vi "Periodic Tasks.vi"(8 "error in":errorcluster) -> ()   [LabVIEW 2016]
doc: "This VI runs in parallel to other tasks. It can contain as many user-defined periodic loops as you need. These can carry out PID or other sorts of timed response."
uses:
  Refname/Motors.ctl
  Refname/Sensors.ctl
  Refname/Queues.ctl
  <vilib>/Rock Robotics/WPI/DriverStation/WPI_DriverStationRobotMode2.ctl
  Refname/Refname to String (Motors).vi
  Robot Global Data.vi
  Refname/Refname to String (Sensors).vi
panel:
  in  "Low Sensitivity z":dbl=1.9 format="%#_13g"
  in  "Default Sensitivity z":dbl=1.6 format="%#_13g"
  in  "Low Sensitivity x & y":dbl=1.7 format="%#_13g"
  in  "Default Sensitivity x & y":dbl=1.4 format="%#_13g"
  out "error out":errorcluster
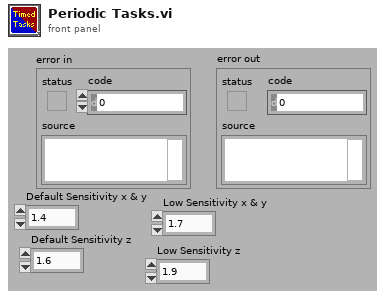
[diagram p1: front panel]
types:
  T1 = typedef "Queues.ctl" = enum16{"Log Queue"}
  T2 = typedef "Sensors.ctl" = enum16{"DIP 1", "DIP 2", "DIP 3", "DIP 4", "IMU", "HuskieBoard"}
  T3 = typedef "Motors.ctl" = enum16{"Wheel 1", "Swerve 1", "Wheel 2", "Swerve 2", "Wheel 3", "Swerve 3", "Wheel 4", "Swerve 4", "Climber"}
  T4 = typedef "WPI_MotorControlDeviceRef.ctl" = cluster{"DeviceStatus":errorcluster, "Type":T5, "PWM":cluster{"PWM Channel":T6, "DeadBand":T7}, "CAN":cluster{"Device Number":u8, "SetOutput VI Ref":variant, "GetOutput VI Ref":variant, "Enable VI Ref":variant, "Disable VI Ref":variant, "Data":variant}, "Invert":bool}
  T5 = typedef "WPI_MotorControlType.ctl" = enum16{"PWM", "CAN"}
  T6 = typedef "FPGA_DIOPWMChannel.ctl" = enum8{"PWM 0", "PWM 1", "PWM 2", "PWM 3", "PWM 4", "PWM 5", "PWM 6", "PWM 7", "PWM 8", "PWM 9", "PWM MXP 0", "PWM MXP 1", "PWM MXP 2", "PWM MXP 3", "PWM MXP 4", "PWM MXP 5", "PWM MXP 6", "PWM MXP 7", "PWM MXP 8", "PWM MXP 9", "Invalid"}
  T7 = typedef "WPI_PWMDeadband.ctl" = cluster{"Name":string, "maxPositivePwm":i32, "minPositivePwm":i32, "centerPwm":i32, "maxNegativePwm":i32, "minNegativePwm":i32, "angularRange":u16}
  T8 = typedef "WPI_SerialPortRef.ctl" = cluster{"DevStatus":errorcluster, "Serial Port Name":refnum<visa-resource-name>}
  T9 = typedef "WPI_DriverStationRobotMode2.ctl" = enum16{"Autonomous Disabled", "Autonomous Enabled", "Teleop Disabled", "Teleop Enabled", "Disconnected", "Finish", "Test Disabled", "Test Enabled", "Emergency Stopped"}
  T10 = cluster{"X":dbl, "Y":dbl, "Z":dbl, "B (Straight Drive)":bool, "T1 (Climber Up)":bool, "T2 (Climber Down)":bool, "Pinky Trigger (Low Sensitivity Drive)":bool, "Trigger Full Press (Reverse Drive)":bool}
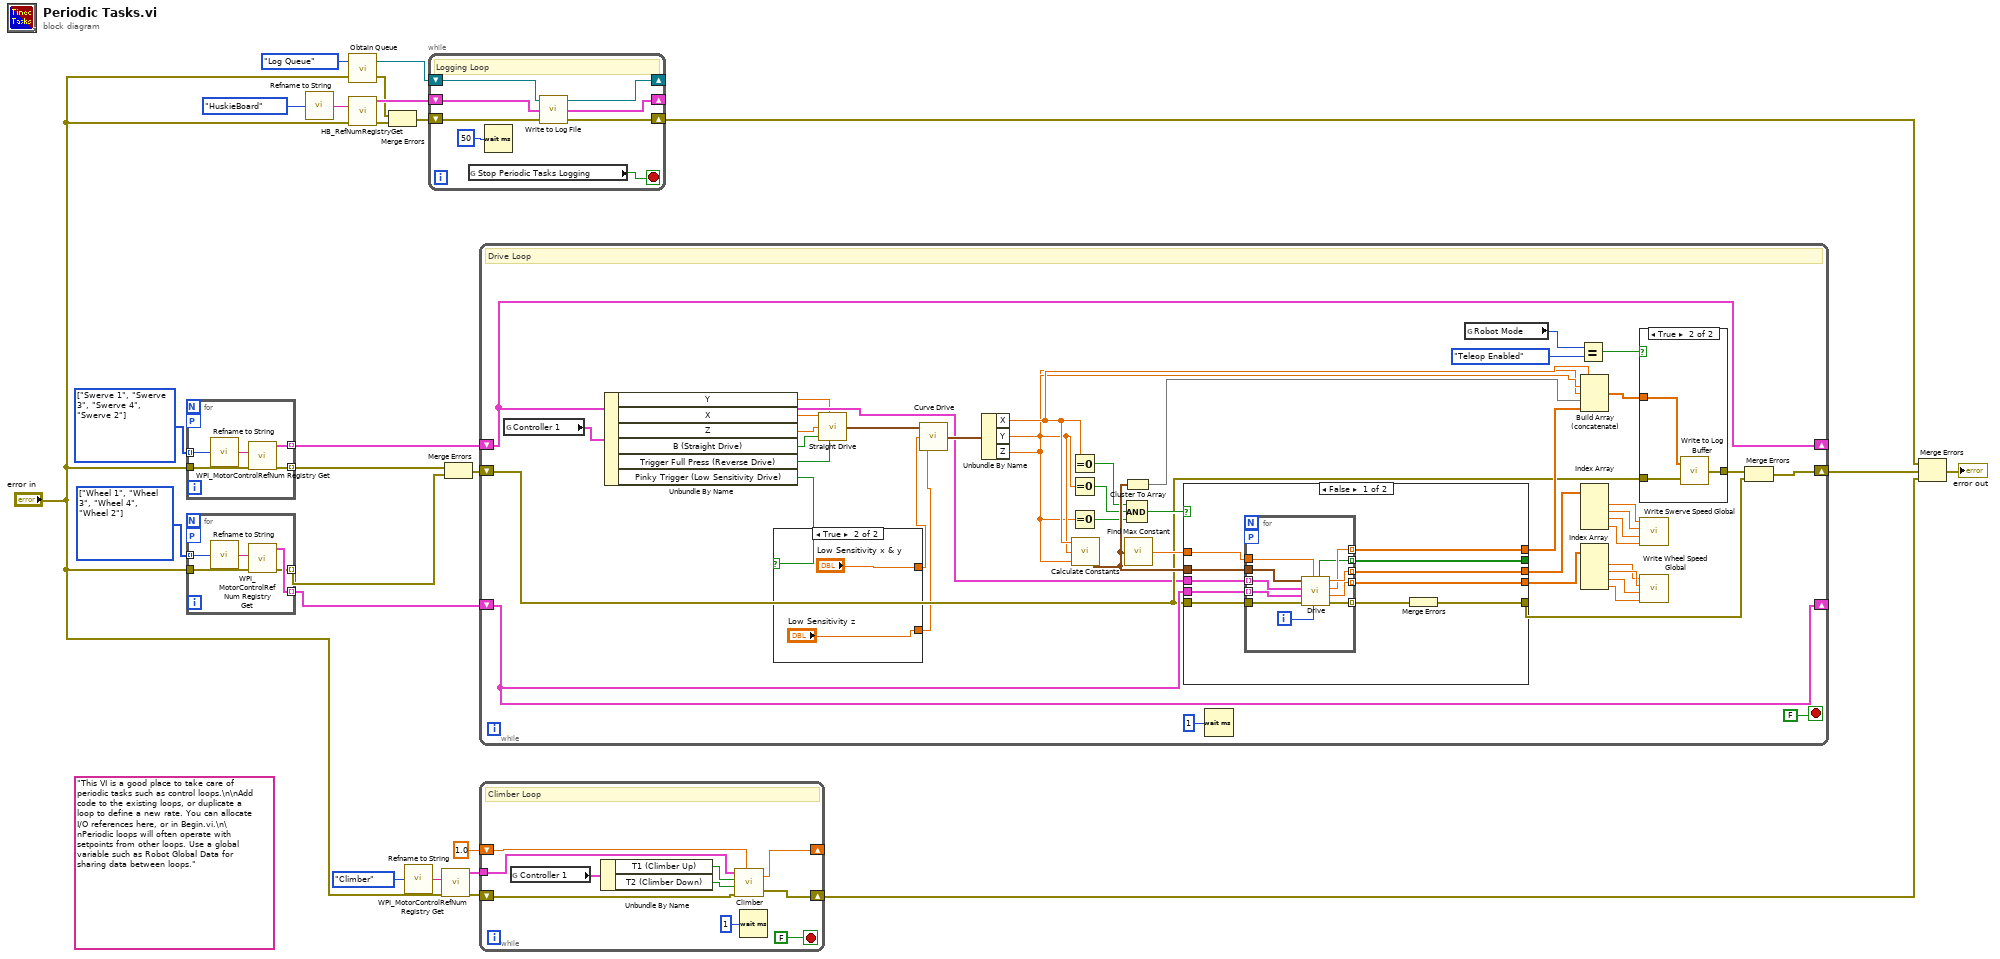
[diagram p0: block diagram]
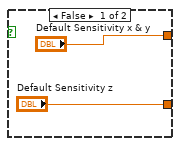
[diagram p2: hidden frame]
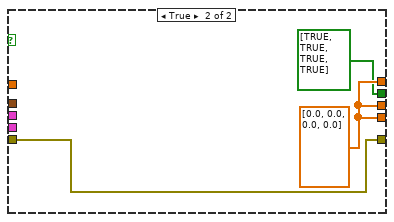
[diagram p3: hidden frame]
diagram:
  w22 = T3[] [enum."Wheel 1", enum."Wheel 3", enum."Wheel 4", enum."Wheel 2"] items=["Wheel 1", "Swerve 1", "Wheel 2", "Swerve 2", "Wheel 3", "Swerve 3", "Wheel 4", "Swerve 4", "Climber"]
  w23 = T3[] [enum."Swerve 1", enum."Swerve 3", enum."Swerve 4", enum."Swerve 2"] items=["Wheel 1", "Swerve 1", "Wheel 2", "Swerve 2", "Wheel 3", "Swerve 3", "Wheel 4", "Swerve 4", "Climber"]
  (unwired) "This VI is a good place to take care of periodic tasks such as control loops.\n\nAdd code to the existing loops, or duplicate a loop to define a new rate. You can allocate I/O references here, or in Begin.vi.\n\nPeriodic loops will often operate with setpoints from other loops. Use a global variable such as Robot Global Data for sharing data between loops."
  n1 = for {
    tunnel: [w30] -> w25 mode=indexing
    tunnel: w23 -> [w28] mode=indexing
    workers-P: _ -> [_]
    tunnel: "error in" -> [w27]
    tunnel: [w26] -> w20 mode=indexing
    n2 = call-poly "Refname to String.vi"("Enum"=w28) -> ("String"=w29:string)
    n3 = call <vilib>:"WPI_MotorControlRefNum Registry Get.vi"("error in (no error)"=w27, "refnum name"=w29) -> ("error out"=w26:errorcluster, "MotorControlDevRef"=w30:T4)  [unwired: 8 in]
  }
  n4 = for {
    tunnel: [w35] -> w24 mode=indexing
    tunnel: w22 -> [w33] mode=indexing
    workers-P: _ -> [_]
    tunnel: "error in" -> [w32]
    tunnel: [w31] -> w19 mode=indexing
    n5 = call-poly "Refname to String.vi"("Enum"=w33) -> ("String"=w34:string)
    n6 = call <vilib>:"WPI_MotorControlRefNum Registry Get.vi"("error in (no error)"=w32, "refnum name"=w34) -> ("error out"=w31:errorcluster, "MotorControlDevRef"=w35:T4)  [unwired: 8 in]
  }
  n7 = call-poly "Refname to String.vi"("Enum"=Sensors."HuskieBoard") -> ("String"=w11:string)
  n8 = call "Obtain Queue.vi"("error in"="error in", "Queue"=Queues."Log Queue") -> ("error out"=w5:errorcluster, "Queue Ref"=w8:refnum<queue>)
  n9 = call <vilib>:"HB_RefNumRegistryGet.vi"("refnum name"=w11, "error in (no error)"="error in") -> ("HBDevRef"=w7:T8, "error out"=w4:errorcluster)  [unwired: 12 in]
  n10 = Merge Errors(w5, w4) -> (w6:errorcluster)
  n11 = call-poly "Refname to String.vi"("Enum"=Motors."Climber") -> ("String"=w18:string)
  n12 = while {
    shift-right: [w41] -> _
    shift-left: w8 -> [w42]
    shift-right: [w39] -> _
    shift-left: w7 -> [w40]
    shift-right: [w37] -> w3
    shift-left: w6 -> [w38]
    stop <- w43 stop-if-true
    # "Logging Loop"
    n13 = global read "Robot Global Data.vi" "Stop Periodic Tasks Logging"() -> (w43:bool)
    n14 = Wait (ms)(milliseconds to wait=u32 50) -> ()  [unwired: 1 out]
    n15 = call "Write to Log File.vi"("error in"=w38, "HBDevRef"=w40, "Log Queue"=w42) -> ("error out"=w37:errorcluster, "HBDevRef"=w39:T8, "Log Queue"=w41:refnum<queue>)
  }
  n16 = call <vilib>:"WPI_MotorControlRefNum Registry Get.vi"("error in (no error)"="error in", "refnum name"=w18) -> ("error out"=w15:errorcluster, "MotorControlDevRef"=w16:T4)  [unwired: 8 in]
  n17 = Merge Errors(w20, w19) -> (w13:errorcluster)
  n18 = while {
    shift-right: [w53] -> _
    shift-left: w25 -> [w53]
    shift-right: [w85] -> _
    shift-left: w24 -> [w85]
    shift-right: [w68] -> w2
    shift-left: w13 -> [w54]
    stop <- FALSE stop-if-true
    # "Drive Loop"
    n19 = global read "Robot Global Data.vi" "Controller 1"() -> (w49:T10)
    n20 = Unbundle By Name(w49) -> ("Y"=w45:dbl, "X"=w44:dbl, "Z"=w46:dbl, "B (Straight Drive)"=w47:bool, "Trigger Full Press (Reverse Drive)"=w48:bool, "Pinky Trigger (Low Sensitivity Drive)"=w52:bool)
    n21 = case shown="True" w52 {
      tunnel: ["Default Sensitivity x & y" "Low Sensitivity x & y"] -> w51
      tunnel: ["Default Sensitivity z" "Low Sensitivity z"] -> w50
      frame False {
      }
      frame True {
      }
    }
    n22 = call "Straight Drive.vi"("X"=w44, "Y"=w45, "Z"=w46, "Straight?"=w47, "Reverse?"=w48) -> ("Axes Magnitudes"=w55:cluster{"X":dbl, "Y":dbl, "Z":dbl})
    n23 = call "Curve Drive.vi"("z exponent"=w50, "x & y exponent"=w51, "Axes Magnitudes"=w55) -> ("Axes Magnitudes"=w56:cluster{"X":dbl, "Y":dbl, "Z":dbl})
    n24 = Unbundle By Name(w56) -> ("X"=w59:dbl, "Y"=w58:dbl, "Z"=w57:dbl)
    n25 = Equal To 0?(x=w59) -> (x = 0?=w76:bool)
    n26 = Equal To 0?(x=w58) -> (x = 0?=w75:bool)
    n27 = Equal To 0?(x=w57) -> (x = 0?=w74:bool)
    n28 = call "Calculate Constants.vi"("Z"=w57, "Y"=w58, "X"=w59) -> ("constants cluster"=w78:cluster{"a":dbl, "b":dbl, "c":dbl, "d":dbl})
    n29 = Cluster To Array(cluster=w78) -> (array=w64:dbl[])
    n30 = call "Find Max Constant.vi"("constants"=w78) -> ("Max or 1"=w77:dbl)
    n31 = Compound Arithmetic op=AND(w76, w75, w74) -> (w73:bool)
    n32 = case shown="False" w73 {
      tunnel: w85 -> [w102 _]
      tunnel: [w101 w116] -> w82
      tunnel: [w100 w116] -> w81
      tunnel: w54 -> [w99 w115]
      tunnel: w53 -> [w98 _]
      tunnel: w78 -> [w97 _]
      tunnel: w77 -> [w96 _]
      tunnel: [w95 w116] -> w65
      tunnel: [w94 w115] -> w60
      tunnel: [w92 bool[] [TRUE, TRUE, TRUE, TRUE]] -> _
      frame False {
        n33 = for {
          tunnel: w98 -> [w104] mode=indexing
          tunnel: w102 -> [w113] mode=indexing
          tunnel: [w112] -> w101 mode=indexing
          tunnel: [w111] -> w100 mode=indexing
          tunnel: w99 -> [w110]
          tunnel: [w106] -> w93 mode=indexing
          tunnel: w97 -> [w109]
          tunnel: w96 -> [w108]
          tunnel: [w105] -> w95 mode=indexing
          workers-P: _ -> [_]
          tunnel: [w103] -> w92 mode=indexing
          i -> [w107]
          n34 = call "Drive.vi"("Index"=w107, "Max Speed or 1"=w108, "error in"=w110, "Wheel DevRef"=w113, "Swerve DevRef"=w104, "constants"=w109) -> ("error out"=w106:errorcluster, "Wheel Speed"=w111:dbl, "Setpoint"=w105:dbl, "Swerve Speed"=w112:dbl, "Reverse?"=w103:bool)  [unwired: 1 in]
        }
        n35 = Merge Errors(w93) -> (w94:errorcluster)
      }
      frame True {
        w116 = dbl[] [0.0, 0.0, 0.0, 0.0]
      }
    }
    n36 = Wait (ms)(milliseconds to wait=u32 1) -> ()  [unwired: 1 out]
    n37 = global read "Robot Global Data.vi" "Robot Mode"() -> (w61:T9)
    n38 = Equal?(x=w61, y=WPI_DriverStationRobotMode2."Teleop Enabled" ("Robot Mode")) -> (x = y?=w63:bool)
    n39 = Build Array (concatenate)(w59, w58, w57, w64, w65) -> (w66:dbl[])
    n40 = Index Array(array=w82) -> (element #1=w72:dbl, element #2=w71:dbl, element #3=w70:dbl, element #4=w69:dbl)  [unwired: 4 in]
    n41 = Index Array(array=w81) -> (element #1=w83:dbl, element #2=w84:dbl, element #3=w80:dbl, element #4=w79:dbl)  [unwired: 4 in]
    n42 = case shown="True" w63 {
      tunnel: w66 -> [_ w118]
      tunnel: [w117 w120] -> w67
      tunnel: w54 -> [w117 w119]
      frame False {
      }
      frame True {
        n43 = call "Write to Log Buffer.vi"("error in"=w119, "array of values"=w118) -> ("error out"=w120:errorcluster)
      }
    }
    n44 = call "Write Swerve Speed Global.vi"("Swerve 4"=w69, "Swerve 3"=w70, "Swerve 2"=w71, "Swerve 1"=w72) -> ()
    n45 = call "Write Wheel Speed Global.vi"("Wheel 4"=w79, "Wheel 3"=w80, "Wheel 2"=w84, "Wheel 1"=w83) -> ()
    n46 = Merge Errors(w67, w60) -> (w68:errorcluster)
  }
  n47 = while {
    tunnel: w16 -> [w126]
    shift-right: [w125] -> _
    shift-left: 1.0 ("Multiplier") -> [w124]
    shift-right: [w121] -> w1
    shift-left: w15 -> [w127]
    stop <- FALSE stop-if-true
    # "Climber Loop"
    n48 = global read "Robot Global Data.vi" "Controller 1"() -> (w130:T10)
    n49 = Unbundle By Name(w130) -> ("T1 (Climber Up)"=w129:bool, "T2 (Climber Down)"=w128:bool)
    n50 = call "Climber.vi"("Climber Dev Ref"=w126, "Forward Climb"=w129, "Backwards Climb"=w128, "error in"=w127, "Current Multiplier"=w124) -> ("Multiplier"=w125:dbl, "error out"=w121:errorcluster)
    n51 = Wait (ms)(milliseconds to wait=u32 1) -> ()  [unwired: 1 out]
  }
  n52 = Merge Errors(w3, w2, w1) -> (→"error out":errorcluster)
